vi "Actor Core.vi"(8 "error in":errorcluster, 11 "Resynchronization in":refnum<class "Resynchronization.lvclass">) -> (0 "error out":errorcluster, 3 "Actor out":refnum<class "Actor.lvclass">)   [LabVIEW 2018, in "Resynchronization Actor.lvlib" / "Resynchronization.lvclass"]
doc: "(<B>Filename</B>: Actor Framework.lvlib:Actor.lvclass:Actor Core.vi)\n\nReceives messages to the actor, reacts to them, and initiates any error handling that may shut the actor down.\n\nDescendant classes may override this VI to append parallel tasks for the actor to complete while it handles messages. Overrides use the Call Parent Method node."
uses:
  Resynchronization.lvclass
  <vilib>/ActorFramework/Actor/Actor.lvclass
  C:/Users/Administrator/Desktop/LabVIEW EMS/EMS Generic Actor/EMS Generic/EMS Generic.lvclass
  C:/Users/Administrator/Desktop/LabVIEW EMS/Optimization/Generic Optimization Actor/Generic Optimization/Generic Optimization.lvclass
  C:/Users/Administrator/Desktop/LabVIEW EMS/Device Communication and Control Abstract Actor/Device Communication and Control Abstract/Device Communication and Control Abstract.lvclass
  Generic Optimization Actor/Generic Optimization/Optimization Controls/PCC Data.ctl
  EMS Generic Actor/EMS Generic/EMS Generic.lvclass/EMS Generic.ctl
  <vilib>/ORNL/CSEISMIC DDS/CSEISMIC DDS Base/Data Types/PCC_Transition.ctl
  <vilib>/ORNL/CSEISMIC DDS/CSEISMIC DDS Base/Data Types/Controls/DeviceID.ctl
  <vilib>/ActorFramework/Actor/Actor.lvclass/Actor.ctl
  Device Communication and Control Abstract Actor/Device Communication and Control Abstract/Device Communication and Control Abstract.lvclass/Device Communication and Control Abstract.ctl
  Device Communication and Control Abstract Actor/Device Communication and Control Abstract Messages/Set PCC Transition Msg/Set PCC Transition Msg.lvclass/Set PCC Transition Msg.ctl
  <vilib>/ActorFramework/Message Enqueuer/Message Enqueuer.lvclass/Message Enqueuer.ctl
  Device Communication and Control Abstract Actor/Device Communication and Control Abstract Messages/Set PCC Transition Msg/Send Set PCC Transition.vi
  <vilib>/ActorFramework/Actor/Read Caller Enqueuer.vi
  <vilib>/ActorFramework/Message Enqueuer/Enqueue.vi
  Device Communication and Control Abstract Actor/Device Communication and Control Abstract/Device Communication and Control Abstract.lvclass
  C:/Program Files (x86)/National Instruments/LabVIEW 2018/vi.lib/ActorFramework/Actor/Actor.lvclass
  Device Communication and Control Abstract Actor/Device Communication and Control Abstract Messages/Set PCC Transition Msg/Set PCC Transition Msg.lvclass
  C:/Program Files (x86)/National Instruments/LabVIEW 2018/vi.lib/ActorFramework/Message/Message.lvclass
  <vilib>/ActorFramework/Message Priority Queue/Priority Enqueue.vi
  Generic Optimization Actor/Generic Optimization/Generic Optimization.lvclass
  <vilib>/ORNL/CSEISMIC DDS/CSEISMIC DDS Base/CSEISMIC DDS.lvclass
  EMS Generic Actor/EMS Generic/EMS Generic.lvclass
  Utilities/Status Messaging.llb/Status Messaging.lvlib
panel:
  out "Solution Result":string="Waiting"
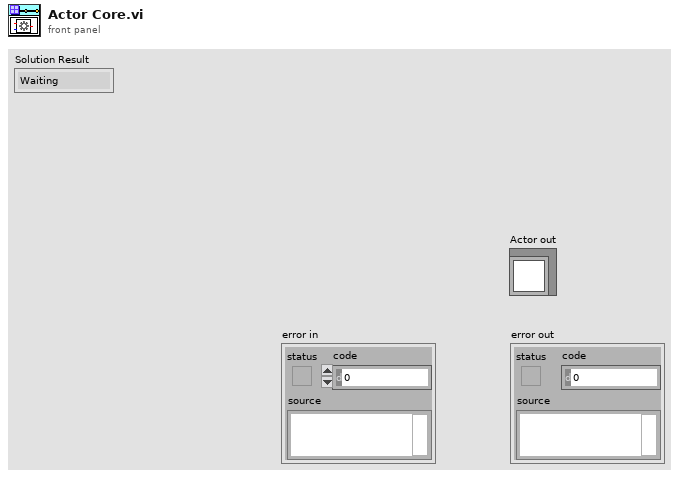
[diagram p1: front panel]
types:
  T1 = typedef "Generic Optimization Actor.lvlib/Generic Optimization.lvclass/PCC Data.ctl" = cluster{"PCC_max":dbl[], "PCC_min":dbl[], "QCC_max":dbl[], "QCC_min":dbl[]}
  T2 = typedef "EMS Generic Actor.lvlib/EMS Generic.lvclass/Global Configuration.ctl" = cluster{"Microgrid ID":u8, "VF Device ID":T3, "Ongrid VF Priority":T3[], "Offgrid VF Priority":T3[], "AutoSwap Offgrid VF":u32, "AutoSwap Offgrid VF Delay (sec)":dbl, "AutoSwap Resynch VF":u32, "PCC Device ID":T3, "Device ID Array":T3[], "Nominal Voltage":dbl, "Nominal Frequency":dbl, "Resynch Timeout (sec)":dbl, "Island VF Activate Timeout (sec)":dbl, "Island PCC Target Power (kW)":dbl, "Island PCC Target Power Timeout (sec)":dbl, "Island Grid Settle Time (sec)":dbl, "Island PCC Failure Timeout (sec)":dbl, "Activation Devices Present Timeout (sec)":dbl, "Activation Devices Activated Timeout (sec)":dbl, "Blackstart VF GenMode Wait (sec)":dbl, "Blackstart VF DERCtrl Wait (sec)":dbl, "Blackstart Success Wait (sec)":dbl, "OnGrid Optimization Delay (sec)":dbl, "OffGrid Optimization Delay (sec)":dbl, "Resynch Frequency (Hz)":dbl, "Optimization Path":string}
  T3 = typedef "CSEISMIC DDS.lvlib/CSEISMIC DDS.lvclass/DeviceID.ctl" = string
  T4 = typedef "Generic Optimization Actor.lvlib/Generic Optimization.lvclass/Bus by ID.ctl" = cluster{"DeviceID":T3, "Bus ID":dbl}
  T5 = typedef "Generic Optimization Actor.lvlib/Generic Optimization.lvclass/Electrical Network Optimization Data.ctl" = cluster{"From_Bus":dbl, "To_Bus":dbl, "Network Resistance":dbl, "Network Reactance":dbl, "Power Flow Limits":dbl[], "Linear Piecewise Power Flow":dbl[], "Reactive Flow Limit":dbl[], "Linear Piecewise Reactive Flow":dbl[]}
  T6 = typedef "CSEISMIC DDS.lvlib/CSEISMIC DDS.lvclass/PCC_Transition.ctl" = cluster{"DeviceID":T3, "Island":bool, "Resynchronize":bool}
  T7 = typedef "CSEISMIC DDS.lvlib/CSEISMIC DDS.lvclass/IED_Status.ctl" = cluster{"DeviceID":T3, "Timestamp":T8, "MicrogridID":u8, "Active":bool, "Inactive":bool, "Error":i32, "Fault":bool, "ErrorString":string}
  T8 = typedef "CSEISMIC DDS.lvlib/CSEISMIC DDS.lvclass/Timestamp.ctl" = cluster{"Seconds":u64, "Remainder":u64}
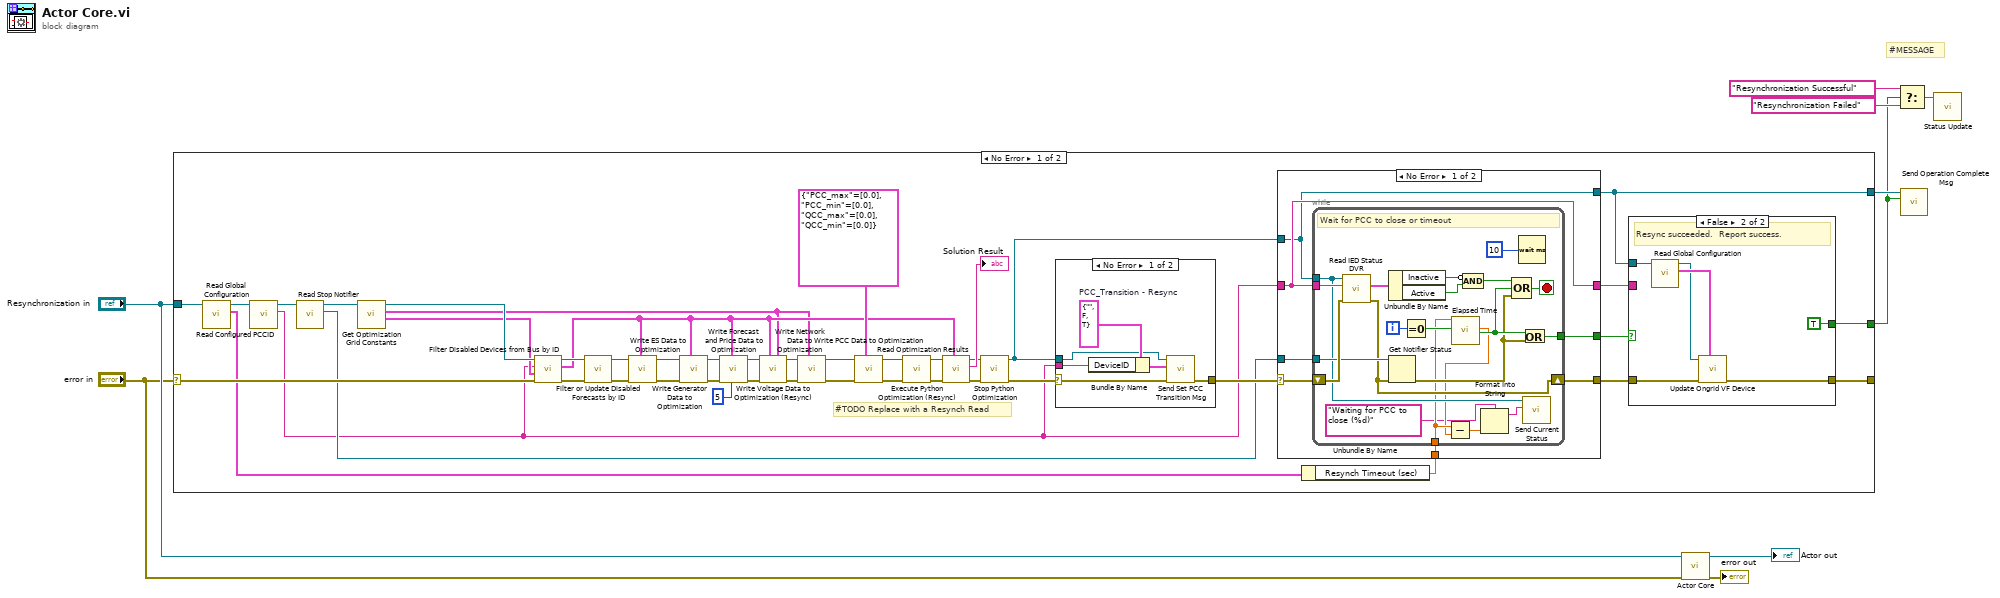
[diagram p0: block diagram]
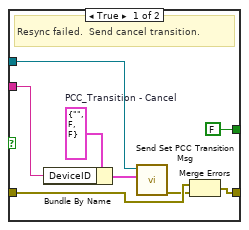
[diagram p2: hidden frame]
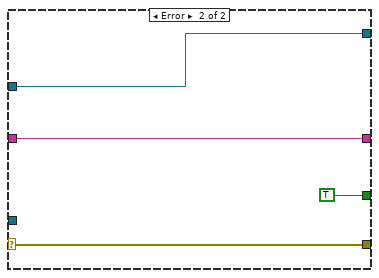
[diagram p3: hidden frame]
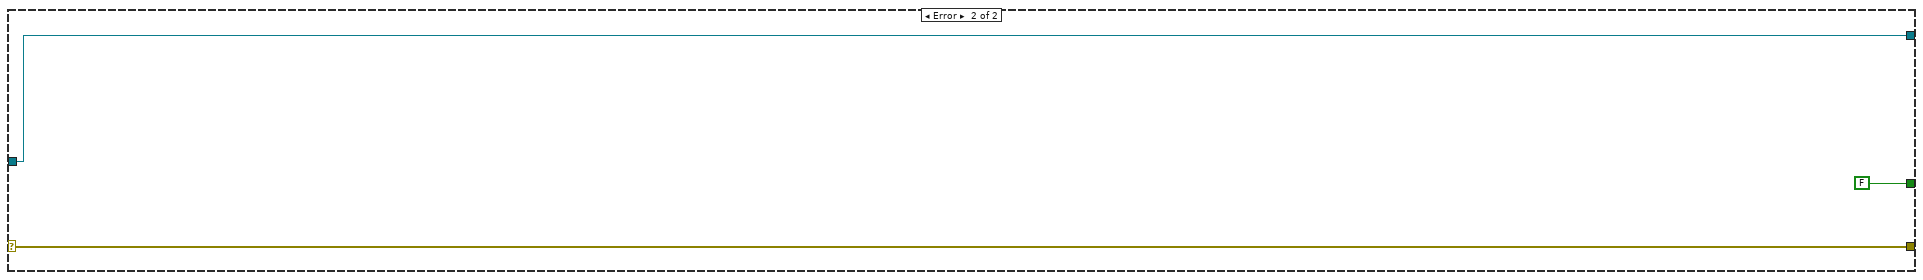
[diagram p5: hidden frame]
diagram:
  # "#MESSAGE"
  n1 = case shown="No Error" "error in" {
    selector: "error in" -> [w30 w108]
    tunnel: "Resynchronization in" -> [w14 w109]
    tunnel: [w18 FALSE] -> w1
    tunnel: [w17 w109] -> w5
    tunnel: [w16 w108] -> _
    frame No Error {
      # "#TODO Replace with a Resynch Read"
      n2 = call "Read Global Configuration.vi"("EMS Generic in"=w14) -> ("Global Configuration"=w12:T2, "dup EMS Generic out"=w13:refnum<class "Resynchronization.lvclass">)  [unwired: 8 in, 1 out]
      n3 = call "Read Configured PCCID.vi"("EMS Generic in"=w13) -> ("PCCID"=w19:T3, "EMS Generic out"=w20:refnum<class "Resynchronization.lvclass">)  [unwired: 8 in, 1 out]
      n4 = call "Read Stop Notifier.vi"("EMS Generic in"=w20) -> ("stop"=w24:refnum<notifier>, "EMS Generic out"=w21:refnum<class "Resynchronization.lvclass">)  [unwired: 9 in]
      n5 = call "Get Optimization Grid Constants.vi"("Generic Optimization in"=w21) -> ("Bus by ID"=w22:T4[], "Network Data"=w10:T5[], "Generic Optimization out"=w23:refnum<class "Resynchronization.lvclass">)  [unwired: 8 in]
      n6 = call "Filter Disabled Devices from Bus by ID.vi"("error in"=w30, "BusData"=w22, "PCCID"=w19, "Generic Optimization in"=w23) -> ("dup error out"=w39:errorcluster, "Filtered Bus by ID"=w34:T4[], "Generic Optimization out"=w40:refnum<class "Resynchronization.lvclass">)  [unwired: 5 in]
      n7 = call "Filter or Update Disabled Forecasts by ID.vi"("error in"=w39, "Generic Optimization in"=w40) -> ("dup error out"=w38:errorcluster, "Generic Optimization out"=w37:refnum<class "Resynchronization.lvclass">)  [unwired: 8 in]
      n8 = call "Write ES Data to Optimization.vi"("Bus by ID"=w34, "error in"=w38, "Generic Optimization in"=w37) -> ("error out"=w54:errorcluster, "Generic Optimization out"=w53:refnum<class "Resynchronization.lvclass">)  [unwired: 7 in]
      n9 = call "Write Generator Data to Optimization.vi"("Bus by ID"=w34, "error in"=w54, "Generic Optimization in"=w53) -> ("error out"=w36:errorcluster, "Generic Optimization out"=w33:refnum<class "Resynchronization.lvclass">)  [unwired: 7 in]
      n10 = call "Write Forecast and Price Data to Optimization.vi"("Max Forecast Length (-1: no limit)"=5, "Bus by ID"=w34, "error in"=w36, "Generic Optimization in"=w33) -> ("error out"=w35:errorcluster, "Generic Optimization out"=w32:refnum<class "Resynchronization.lvclass">)  [unwired: 6 in]
      n11 = call "Write Voltage Data to Optimization (Resync).vi"("Network Data Array"=w10, "Bus by ID"=w34, "error in"=w35, "Generic Optimization in"=w32) -> ("error out"=w42:errorcluster, "Generic Optimization out"=w41:refnum<class "Resynchronization.lvclass">)  [unwired: 6 in]
      n12 = call "Write Network Data to Optimization.vi"("Network Data Array"=w10, "error in"=w42, "Generic Optimization in"=w41) -> ("error out"=w46:errorcluster, "Generic Optimization out"=w47:refnum<class "Resynchronization.lvclass">)  [unwired: 7 in]
      n13 = call "Write PCC Data to Optimization.vi"("PCC Data"=T1 {"PCC_max"=[0.0], "PCC_min"=[0.0], "QCC_max"=[0.0], "QCC_min"=[0.0]}, "error in"=w46, "Generic Optimization in"=w47) -> ("error out"=w45:errorcluster, "Generic Optimization out"=w44:refnum<class "Resynchronization.lvclass">)  [unwired: 7 in]
      n14 = call "Execute Python Optimization (Resync).vi"("error in"=w45, "Resynchronization in"=w44) -> ("error out"=w50:errorcluster, "Resynchronization out"=w51:refnum<class "Resynchronization.lvclass">)  [unwired: 8 in]
      n15 = call "Read Optimization Results.vi"("Bus by ID Array"=w34, "error in"=w50, "Generic Optimization in"=w51) -> ("error out"=w48:errorcluster, "Solution Result"=→"Solution Result":string, "Generic Optimization out"=w49:refnum<class "Resynchronization.lvclass">)  [unwired: 6 in]
      n16 = call "Stop Python Optimization.vi"("error in"=w48, "Generic Optimization in"=w49) -> ("error out"=w29:errorcluster, "Generic Optimization out"=w15:refnum<class "Resynchronization.lvclass">)  [unwired: 8 in]
      n17 = case shown="No Error" w29 {
        selector: w29 -> [w104 w107]
        tunnel: [w103 w107] -> w28
        tunnel: w19 -> [w102 _]
        tunnel: w15 -> [w101 _]
        frame No Error {
          w105 = T6 {"DeviceID"="", "Island"=FALSE, "Resynchronize"=TRUE}  # PCC_Transition - Resync
          n18 = Bundle By Name(cluster=w105, "DeviceID"=w102) -> (w106:T6)
          n19 = call "Send Set PCC Transition Msg.vi"("error in"=w104, "PCC_Transition"=w106, "SCADA Sub Abstract in"=w101) -> ("error out"=w103:errorcluster)  [unwired: 7 in, 1 out]
        }
        frame Error {
        }
      }
      n20 = Unbundle By Name(w12) -> ("Resynch Timeout (sec)"=w11:dbl)
      n21 = case shown="No Error" w28 {
        selector: w28 -> [w75 w100]
        tunnel: w24 -> [w74 _]
        tunnel: w19 -> [w71 w97]
        tunnel: w15 -> [w70 w98]
        tunnel: [w73 TRUE] -> w26
        tunnel: [w72 w100] -> w27
        tunnel: [w70 w98] -> w17
        tunnel: [w71 w97] -> w25
        tunnel: w11 -> [w69 _]
        frame No Error {
          n22 = while {
            tunnel: w70 -> [w81]
            tunnel: w71 -> [w92]
            shift-right: [w82] -> w72
            shift-left: w75 -> [w90]
            tunnel: w74 -> [w89]
            tunnel: [w87] -> w73
            tunnel: w69 -> [w80]
            i -> [w94]
            stop <- w96 stop-if-true
            # "Wait for PCC to close or timeout"
            n23 = call "Read IED Status DVR.vi"("error in"=w90, "DeviceID"=w92, "EMS Generic in"=w81) -> ("error out"=w82:errorcluster, "IED_Status"=w91:T7)  [unwired: 5 in, 2 out]
            n24 = Unbundle By Name(w91) -> ("Inactive"=w86:bool, "Active"=w85:bool)
            n25 = Get Notifier Status(notifier=w89, error in (no error)=w82) -> (error out=w83:errorcluster)  [unwired: 4 out]
            n26 = Equal To 0?(x=w94) -> (x = 0?=w93:bool)
            n27 = call "Elapsed Time"("Time Target (s)"=w80, "Reset"=w93) -> ("Elapsed Time (s)"=w79:dbl, "Time has Elapsed"=w88:bool)  [unwired: 10 in, 6 out]
            n28 = Subtract(x=w80, y=w79) -> (x-y=w78:dbl)
            n29 = Compound Arithmetic op=AND(invert w86, w85) -> (w84:bool)
            n30 = Format Into String(format string="Waiting for PCC to close (%d)", w78) -> (resulting string=w76:string)  [unwired: 2 in, 1 out]
            n31 = Compound Arithmetic op=OR(w84, w88, w83) -> (w96:bool)
            n32 = Wait (ms)(milliseconds to wait=u32 10) -> ()  [unwired: 1 out]
            n33 = Or(x=w88, y=w83) -> (x .or. y?=w87:bool)
            n34 = call "Send Current Status.vi"("Current Status"=w76, "Device Communication and Control Abstract in"=w81) -> ()  [unwired: 8 in, 2 out]
          }
        }
        frame Error {
        }
      }
      n35 = case shown="False" w26 {
        tunnel: w17 -> [w62 w65]
        tunnel: [w56 w66] -> w16
        tunnel: w25 -> [w60 _]
        tunnel: [FALSE TRUE] -> w18
        tunnel: w27 -> [w57 w67]
        frame True {
          w61 = T6 {"DeviceID"="", "Island"=FALSE, "Resynchronize"=FALSE}  # PCC_Transition - Cancel
          # "Resync failed.  Send cancel transition."
          n36 = Bundle By Name(cluster=w61, "DeviceID"=w60) -> (w59:T6)
          n37 = call "Send Set PCC Transition Msg.vi"("PCC_Transition"=w59, "SCADA Sub Abstract in"=w62) -> ("error out"=w55:errorcluster)  [unwired: 8 in, 1 out]
          n38 = Merge Errors(w57, w55) -> (w56:errorcluster)
        }
        frame False {
          # "Resync succeeded.  Report success."
          n39 = call "Read Global Configuration.vi"("EMS Generic in"=w65) -> ("Global Configuration"=w64:T2, "dup EMS Generic out"=w63:refnum<class "Resynchronization.lvclass">)  [unwired: 8 in, 1 out]
          n40 = call "Update Ongrid VF Device.vi"("Global Configuration"=w64, "error in"=w67, "Resynchronization in"=w63) -> ("error out"=w66:errorcluster)  [unwired: 7 in, 1 out]
        }
      }
    }
    frame Error {
    }
  }
  n41 = call-parent "Actor Core.vi"("error in"="error in", "Actor in"="Resynchronization in") -> ("error out"=→"error out":errorcluster, "Actor out"=→"Actor out":refnum<class "Actor.lvclass">)  [unwired: 8 in]
  n42 = Select(t="Resynchronization Successful", s=w1, f="Resynchronization Failed") -> (s? t:f=w2:string)
  n43 = call "Send Operation Complete Msg.vi"("Operation Complete"=w1, "Generic Optimization in"=w5) -> ()  [unwired: 8 in, 2 out]
  n44 = call "Status Update.vi"("Status Update"=w2) -> ()  [unwired: 9 in, 2 out]
